vi "GetPosSingleAxis.vi"(8 "error in (no error)":errorcluster, 10 "Axis":i32=1 min=1 max=4, 11 "DLOwis in":refnum<class "DLOwis.lvclass">) -> (0 "error out":errorcluster, 2 "Pos":dbl, 3 "DLOwis out":refnum<class "DLOwis.lvclass">)   [LabVIEW 2019, in "DLOwis.lvclass"]
uses:
  DLOwis.lvclass
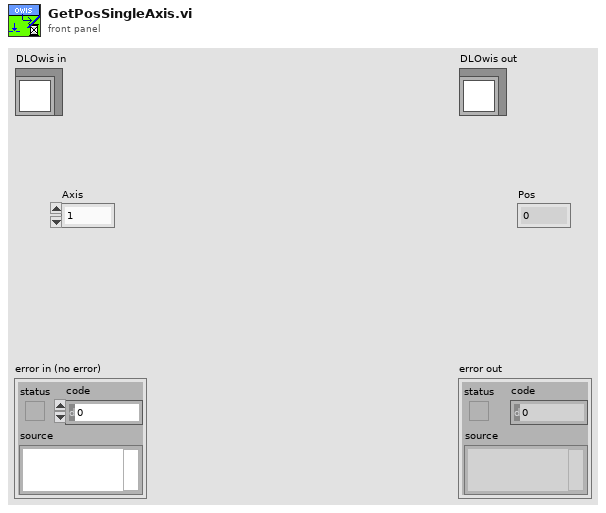
[diagram p1: front panel]
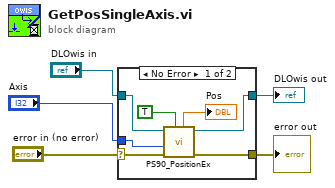
[diagram p0: block diagram]
diagram:
  n1 = case shown="No Error" "error in (no error)" {
    selector: "error in (no error)" -> [w9 w14]
    tunnel: [w7 w14] -> w2
    tunnel: [w11 w13] -> w4
    tunnel: "DLOwis in" -> [w8 w13]
    tunnel: "Axis" -> [w10 _]
    frame No Error {
      n2 = call "PS90_PositionEx.vi"("read?"=TRUE, "error in (no error)"=w9, "Axis number"=w10, "DLOwis.lvclass"=w8) -> ("error out"=w7:errorcluster, "DLOwis.lvclass"=w11:refnum<class "DLOwis.lvclass">, "dValue-Out"=→"Pos":dbl)  [unwired: 4 in]
    }
    frame Error {
    }
  }
  "error out" <- w2
  "DLOwis out" <- w4
